vi "Delete Load Reference VIs.vi"   [LabVIEW 2015]
uses:
  Project Manipulation Scripts/Project Manipulation Scripts.lvlib
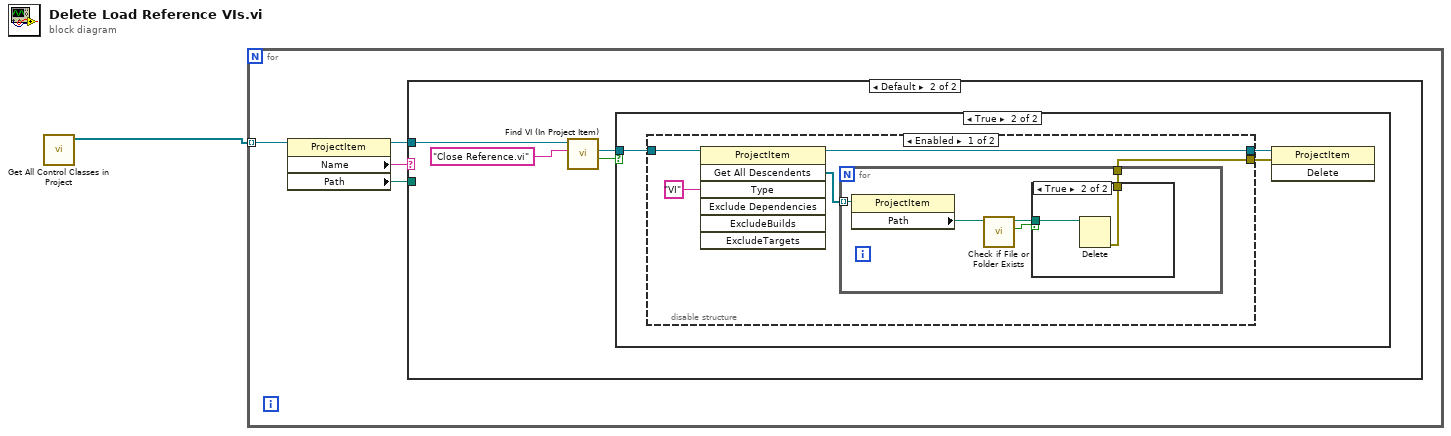
[diagram p0: block diagram]
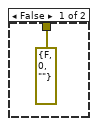
[diagram p4: hidden frame]
diagram:
  n1 = call "Get All Control Classes in Project.vi"() -> ("All Control Classes"=w1:refnum<vi>[])  [unwired: 11 in]
  n2 = for {
    tunnel: w1 -> [w5] mode=indexing
    n3 = property class="ProjectItem"(reference=w5) -> (reference out=w3:refnum<vi>, "Name"=w4:string, "Path"=w2:path)  [unwired: 1 in, 1 out]
    n4 = case shown="Default" w4 {
      tunnel: w3 -> [_ w9]
      tunnel: w2 -> [_ _]
      frame "GObject.lvclass", "Generic.lvclass" {
      }
      frame Default {
        n5 = call "Find VI (In Project Item).vi"("VI Name"="Close Reference.vi" ("format string"), "ProjectItem in"=w9) -> ("Found?"=w7:bool, "VI ProjectItem Refnum"=w8:refnum<vi>)  [unwired: 7 in, 1 out]
        n6 = case shown="True" w7 {
          tunnel: w8 -> [_ w12]
          frame False {
          }
          frame True {
            n7 = disable-structure shown="Enabled" {
              disable-tunnel: w12 -> [w17 w26]
              disable-tunnel: [w16 w26] -> w11
              disable-tunnel: [w15 _] -> w10
              frame Enabled {
                n8 = invoke class="ProjectItem" method="Get All Descendents"(reference=w17, "Type"="VI") -> (reference out=w16:refnum<vi>, "All Descendents"=w14:refnum<vi>[])  [unwired: 5 in, 5 out]
                n9 = for {
                  tunnel: w14 -> [w22] mode=indexing
                  tunnel: [w21] -> w15
                  n10 = property class="ProjectItem"(reference=w22) -> ("Path"=w20:path)  [unwired: 1 in, 2 out]
                  n11 = call <vilib>:"Check if File or Folder Exists.vi"("path"=w20) -> ("file or folder exists?"=w18:bool, "dup path"=w19:path)  [unwired: 8 in, 1 out]
                  n12 = case shown="True" w18 {
                    tunnel: [errorcluster {"status"=FALSE, "code"=0, "source"=""} ("error out") w25] -> w21
                    tunnel: w19 -> [_ w24]
                    frame False {
                    }
                    frame True {
                      n13 = Delete(path (use dialog)=w24) -> (error out=w25:errorcluster)  [unwired: 4 in, 2 out]
                    }
                  }
                }
              }
              frame Disabled {
              }
            }
            n14 = invoke class="ProjectItem" method="Delete"(reference=w11, error in=w10) -> ()  [unwired: 1 in, 3 out]
          }
        }
      }
    }
  }
